vi "Meter Detection GUID Lookup.vi"() -> ()   [LabVIEW 2011, in "Meter Detection Custom Device.lvlib"]
doc: "Use this Global VI to access the GUIDs assigned to the page resources of the Custom Device."
uses:
  Meter Detection Custom Device.lvlib
panel:
  in  "Current Time":string="8acdcb93-8529-42b6-92bf-d443b1dd904b"
  in  "Execution Time":string="66ed530f-2669-461e-b2f5-508ee9997e74"
  in  "Meter Value":string="25dc664e-5f40-4994-9a12-523fe15305a2"
  in  "Custom Device":string="8abc71e6-051e-4bd8-bbb5-f60492892749"
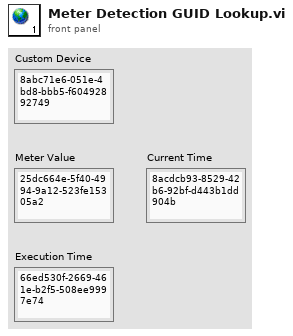
[diagram p1: front panel]
diagram:
